vi "Configure Power Sensor Zeroing.vi"(8 "error in (no error)":errorcluster, 10 "Instance (1)":i32=1 format="%.0g", 11 "VISA resource name":refnum<visa-resource-name>) -> (0 "error out":errorcluster, 3 "VISA resource name out":refnum<visa-resource-name>)   [LabVIEW 2020, in "Rohde&Schwarz CMXP GPRF.lvlib"]
doc: "Initiate zeroing of the power sensor or reads the zeroing state. A running external power sensor measurement is interrupted and re-started after the zeroing procedure has been completed.\n\nAttribute:\nRSCMXPGPRF_ATTR_SENSOR_MEASUREMENT_ZEROING\n\nRemote-control command:\nCALibration:GPRF:MEAS<i>:EPSensor:ZEROing"
uses:
  <instrlib>/Rohde&Schwarz CMXP GPRF/Rohde&Schwarz CMXP GPRF.lvlib
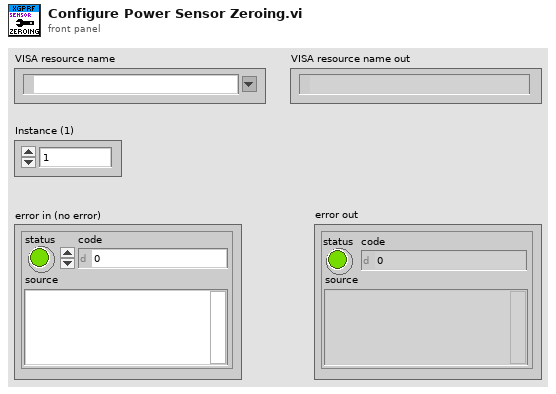
[diagram p1: front panel]
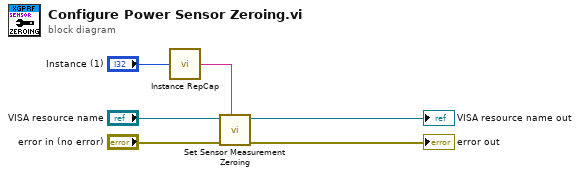
[diagram p0: block diagram]
diagram:
  n1 = call <instrlib>:"Instance RepCap.vi"("Instance in"="Instance (1)") -> ("Instance out"=w6:string)
  n2 = call "Set Sensor Measurement Zeroing"("Repeated Capabilities"=w6, "error in (no error)"="error in (no error)", "instrument handle"="VISA resource name") -> ("error out"=→"error out":errorcluster, "instrument handle out"=→"VISA resource name out":refnum<visa-resource-name>)  [unwired: 7 in]
